vi "DownsampleStage2_5782_10MHzPID.vi"(8 "valid in":bool, 9 "reset":bool, 11 "Data in":fxp<+/-,16,14>[](array[numeric])=[0.0, 0.0, 0.0, 0.0, 0.0, 0.0]) -> (0 "valid out":bool, 3 "data out":fxp<+/-,16,14>[](array[numeric]))   [LabVIEW 2013]
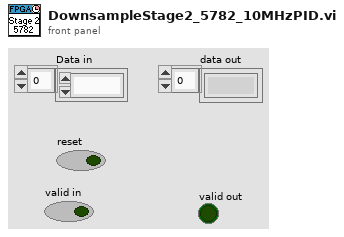
[diagram p1: front panel]
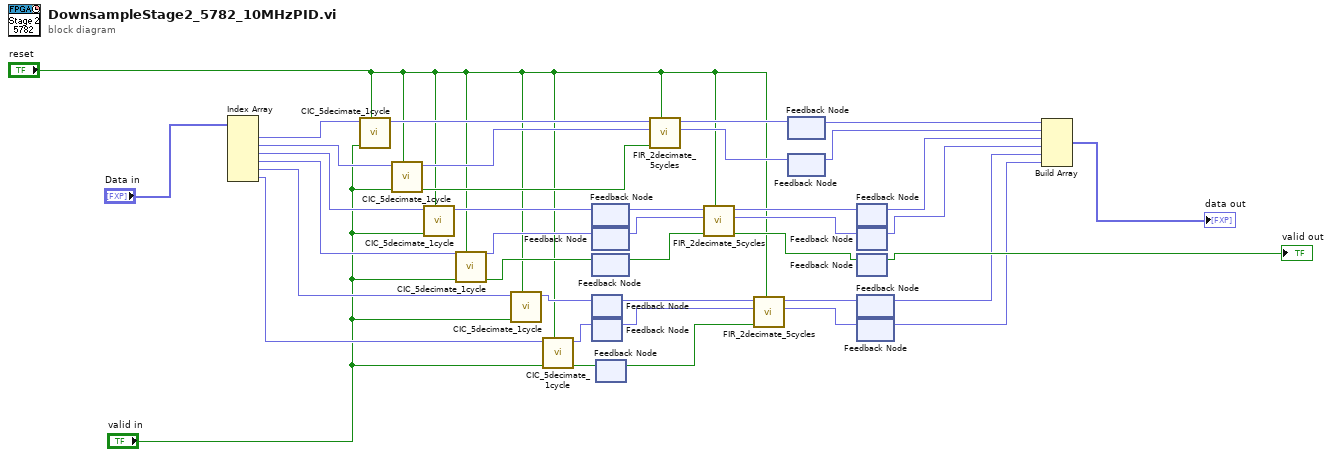
[diagram p0: block diagram]
diagram:
  n1 = Index Array(array="Data in") -> (element #1=w37:fxp<+/-,16,14>, element #2=w35:fxp<+/-,16,14>, element #3=w34:fxp<+/-,16,14>, element #4=w33:fxp<+/-,16,14>, element #5=w14:fxp<+/-,16,14>, element #6=w13:fxp<+/-,16,14>)  [unwired: 6 in]
  n2 = call "CIC_5decimate_1cycle.vi"("reset"="reset", "valid in"="valid in", "Data in"=w37) -> ("Data out"=w26:fxp<+/-,16,14>)  [unwired: 7 in, 1 out]
  n3 = call "CIC_5decimate_1cycle.vi"("reset"="reset", "valid in"="valid in", "Data in"=w35) -> ("valid out"=w24:bool, "Data out"=w25:fxp<+/-,16,14>)  [unwired: 7 in]
  n4 = call "CIC_5decimate_1cycle.vi"("reset"="reset", "valid in"="valid in", "Data in"=w34) -> ("Data out"=w32:fxp<+/-,16,14>)  [unwired: 7 in, 1 out]
  n5 = call "CIC_5decimate_1cycle.vi"("reset"="reset", "valid in"="valid in", "Data in"=w33) -> ("valid out"=w30:bool, "Data out"=w31:fxp<+/-,16,14>)  [unwired: 7 in]
  n6 = call "CIC_5decimate_1cycle.vi"("reset"="reset", "valid in"="valid in", "Data in"=w14) -> ("Data out"=w8:fxp<+/-,16,14>)  [unwired: 7 in, 1 out]
  n7 = call "CIC_5decimate_1cycle.vi"("reset"="reset", "valid in"="valid in", "Data in"=w13) -> ("valid out"=w3:bool, "Data out"=w7:fxp<+/-,16,14>)  [unwired: 7 in]
  n8 = feedback #1() -> (w29:fxp<+/-,16,14>)  [unwired: 1 in]
  n9 = feedback-in #1(w32) -> ()
  n10 = feedback #2() -> (w28:fxp<+/-,16,14>)  [unwired: 1 in]
  n11 = feedback-in #2(w31) -> ()
  n12 = feedback #3() -> (w27:bool)  [unwired: 1 in]
  n13 = feedback-in #3(w30) -> ()
  n14 = feedback #4() -> (w9:fxp<+/-,16,14>)  [unwired: 1 in]
  n15 = feedback-in #4(w8) -> ()
  n16 = feedback #5() -> (w10:fxp<+/-,16,14>)  [unwired: 1 in]
  n17 = feedback-in #5(w7) -> ()
  n18 = feedback #6() -> (w2:bool)  [unwired: 1 in]
  n19 = feedback-in #6(w3) -> ()
  n20 = call "FIR_2decimate_5cycles.vi"("reset"="reset", "valid in"=w24, "Q in"=w25, "I in"=w26) -> ("Q out"=w22:fxp<+/-,16,14>, "I out"=w23:fxp<+/-,16,14>)  [unwired: 4 in, 2 out]
  n21 = call "FIR_2decimate_5cycles.vi"("reset"="reset", "valid in"=w27, "Q in"=w28, "I in"=w29) -> ("valid out"=w17:bool, "Q out"=w18:fxp<+/-,16,14>, "I out"=w19:fxp<+/-,16,14>)  [unwired: 4 in, 1 out]
  n22 = call "FIR_2decimate_5cycles.vi"("reset"="reset", "valid in"=w2, "Q in"=w10, "I in"=w9) -> ("Q out"=w12:fxp<+/-,16,14>, "I out"=w11:fxp<+/-,16,14>)  [unwired: 4 in, 2 out]
  n23 = feedback #7() -> (w21:fxp<+/-,16,14>)  [unwired: 1 in]
  n24 = feedback-in #7(w23) -> ()
  n25 = feedback #8() -> (w20:fxp<+/-,16,14>)  [unwired: 1 in]
  n26 = feedback-in #8(w22) -> ()
  n27 = feedback #9() -> (w15:fxp<+/-,16,14>)  [unwired: 1 in]
  n28 = feedback-in #9(w19) -> ()
  n29 = feedback #10() -> (w16:fxp<+/-,16,14>)  [unwired: 1 in]
  n30 = feedback-in #10(w18) -> ()
  n31 = feedback #11() -> (→"valid out":bool)  [unwired: 1 in]
  n32 = feedback-in #11(w17) -> ()
  n33 = feedback #12() -> (w5:fxp<+/-,16,14>)  [unwired: 1 in]
  n34 = feedback-in #12(w11) -> ()
  n35 = feedback #13() -> (w4:fxp<+/-,16,14>)  [unwired: 1 in]
  n36 = feedback-in #13(w12) -> ()
  n37 = Build Array(w21, w20, w15, w16, w5, w4) -> (→"data out":fxp<+/-,16,14>[])
